vi "Format InstanceStateType_LVXML.vi"(8 "error in (no error)":errorcluster, 10 "xmlData":T2, 11 "AWS_EC2 in":refnum<class "AWS_EC2.lvclass">) -> (0 "error out":errorcluster, 2 "InstanceStateType":T3, 3 "AWS_EC2 out":refnum<class "AWS_EC2.lvclass">)   [LabVIEW 2014, in "AWS_EC2.lvlib" / "AWS_EC2.lvclass"]
uses:
  AWS_EC2.lvclass
  EC2 Datatypes/InstanceStateType.ctl
  lv-xml-parser/r0/trunk/VI Source/EventType.ctl
  AWS_EC2.lvlib
  lv-xml-parser/r0/trunk/VI Source/LV XML Parser.lvlib
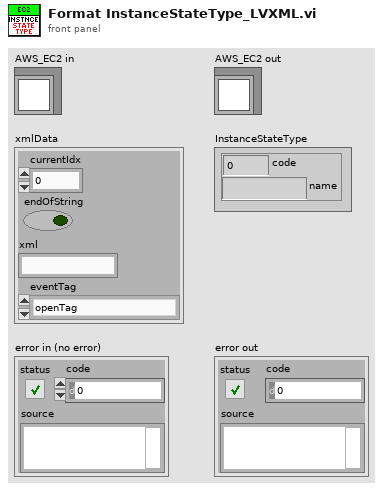
[diagram p1: front panel]
types:
  T1 = typedef "LV XML Parser.lvlib/EventType.ctl" = enum16{"openTag", "endOpenTag", "closeTag", "comment", "endComment", "endOfFile", "attribute", "startXml"}
  T2 = cluster{"currentIdx":i32, "endOfString":bool, "xml":string, "eventTag":T1}
  T3 = typedef "AWS_EC2.lvlib/InstanceStateType.ctl" = cluster{"code":i16, "name":string}
  T4 = cluster{"namespaceUri":string, "localName":string}
  T5 = cluster{"Attributes":cluster{"localName":string, "namespaceUri":string, "value":string}[], "localName":string, "namespaceUri":string, "valueXmlData":cluster{"currentIdx":i32, "endOfString":bool, "xml":string, "eventTag":T1}}[]
  T6 = cluster{"Attributes":cluster{"localName":string, "namespaceUri":string, "value":string}[], "localName":string, "namespaceUri":string, "valueXmlData":cluster{"currentIdx":i32, "endOfString":bool, "xml":string, "eventTag":T1}}
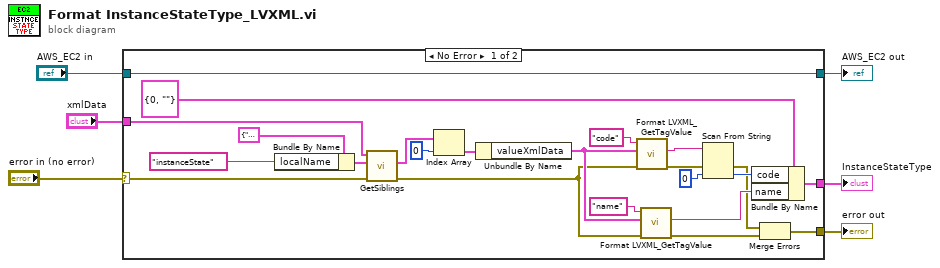
[diagram p0: block diagram]
diagram:
  n1 = case shown="No Error" "error in (no error)" {
    selector: "error in (no error)" -> [w9 w30]
    tunnel: "xmlData" -> [w11 _]
    tunnel: "AWS_EC2 in" -> [w10 w31]
    tunnel: [w10 w31] -> w4
    tunnel: [w8 w30] -> w5
    tunnel: [w7 _] -> w6
    frame No Error {
      n2 = Bundle By Name(cluster=T4 {"namespaceUri"="", "localName"=""} ("limitToTag"), "localName"="instanceState" ("Tag name")) -> (w28:T4)
      n3 = call "GetSiblings.vi"("error in (no error)"=w9, "limitToTag"=w28, "xmlData"=w11) -> ("error out"=w14:errorcluster, "Siblings"=w27:T5)  [unwired: 7 in]
      n4 = Index Array(array=w27, index=0) -> (element=w23:T6)
      n5 = Unbundle By Name(w23) -> ("valueXmlData"=w15:T2)
      n6 = call "Format LVXML_GetTagValue.vi"("error in (no error)"=w14, "xmlDataIn"=w15, "Tag name"="code") -> ("error out"=w19:errorcluster, "Value"=w20:string)  [unwired: 6 in, 1 out]
      n7 = call "Format LVXML_GetTagValue.vi"("error in (no error)"=w14, "xmlDataIn"=w15, "Tag name"="name") -> ("error out"=w12:errorcluster, "Value"=w17:string)  [unwired: 6 in, 1 out]
      n8 = Scan From String(input string=w20, error in=w19, default 1=i16 0 ("code")) -> (error out=w13:errorcluster, output 1=w18:i16)  [unwired: 2 in, 2 out]
      n9 = Bundle By Name(cluster=T3 {"code"=0, "name"=""} ("InstanceStateType"), "code"=w18, "name"=w17) -> (w7:T3)
      n10 = Merge Errors(w13, w12) -> (w8:errorcluster)
    }
    frame Error {
    }
  }
  "InstanceStateType" <- w6
  "error out" <- w5
  "AWS_EC2 out" <- w4
